vi "BSTPassFailTest.vi"() -> (0 "error out":errorcluster, 1 "Report Text":string, 2 "PASS/FAIL Flag":bool=TRUE)   [LabVIEW 2013]
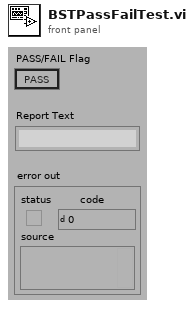
[diagram p1: front panel]
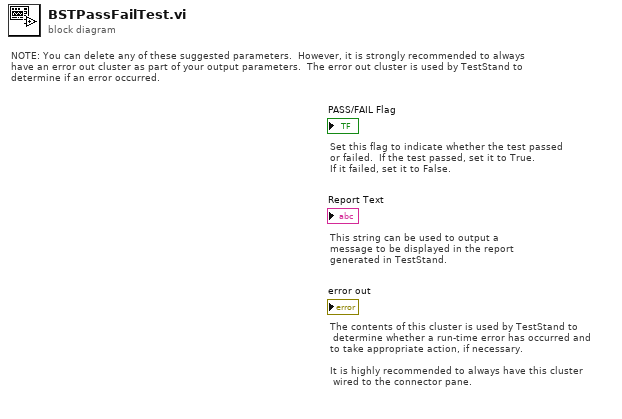
[diagram p0: block diagram]
diagram:
  # "NOTE: You can delete any of these suggested parameters.  However, it is strongly recommended to always have an error out cluster as part of your output parameters.  The error out cluster is used by TestStand to determine if an error occurred."
  # "Set this flag to indicate whether the test passed\nor failed.  If the test passed, set it to True.\nIf it failed, set it to False."
  # "This string can be used to output a\nmessage to be displayed in the report\ngenerated in TestStand."
  # "The contents of this cluster is used by TestStand to\n determine whether a run-time error has occurred and\nto take appropriate action, if necessary.\n\nIt is highly recommended to always have this cluster\n wired to the connector pane."
